vi "Test Overrides Has Case Structure Removed.vi"(8 "error in (no error)":errorcluster, 11 "Test Case In":refnum<class "Pure Mock Class Generator Test.lvclass">) -> (0 "error out":errorcluster, 3 "Test Case Out":refnum<class "Pure Mock Class Generator Test.lvclass">)   [LabVIEW 2020, in "Pure Mock Class Generator Test.lvclass"]
uses:
  Pure Mock Class Generator Test.lvclass
  C:/Program Files (x86)/National Instruments/LabVIEW 2020/vi.lib/Astemes/LUnit/Test Case.lvclass
  <vilib>/Utility/traverseref.llb/TRef TravTarget.ctl
  <vilib>/Astemes/LUnit/Test Case.lvclass/Test Case.ctl
  <vilib>/Astemes/LUnit/Append Fail Result.vi
  <vilib>/Astemes/LUnit/Append Pass Result.vi
  <vilib>/Utility/traverseref.llb/VI Scripting - Traverse.lvlib
  <vilib>/Astemes/LUnit/Test Case.lvclass
  source/Scripting/Pure Mock Class Generator/Pure Mock Class Generator.lvclass
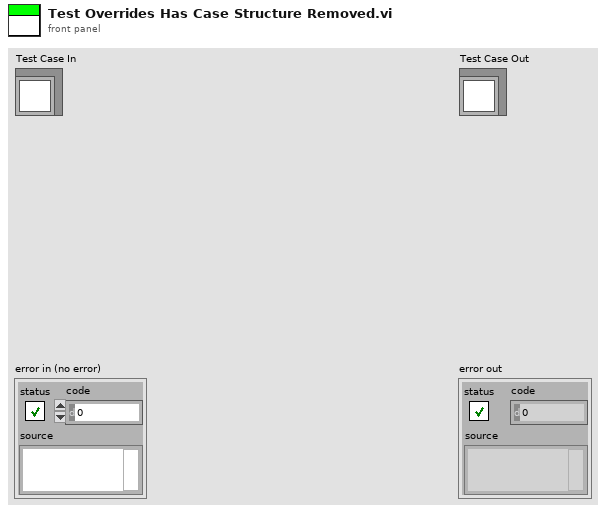
[diagram p1: front panel]
types:
  T1 = typedef "TRef TravTarget.ctl" = enum16{"FP", "BD", "Other"}
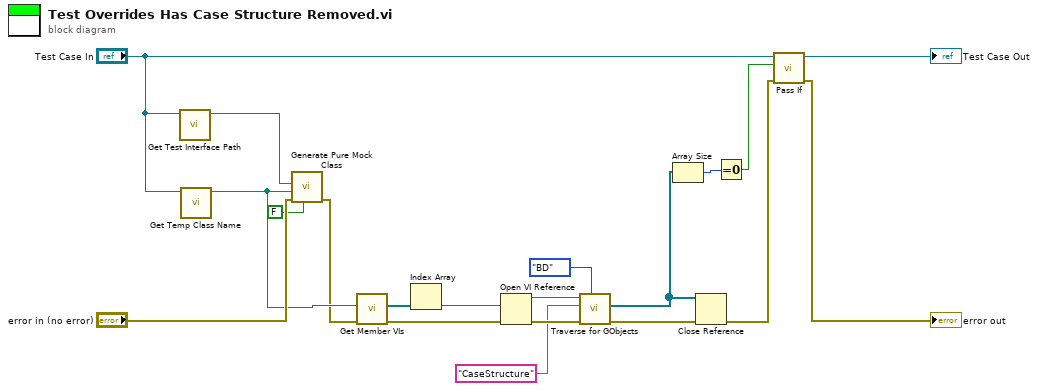
[diagram p0: block diagram]
diagram:
  n1 = call "Get Test Interface Path.vi"("Mock Class Generator Test in"="Test Case In") -> ("Test Class Path"=w16:path)  [unwired: 10 in]
  n2 = call "Get Temp Class Name.vi"("Mock Class Generator Test in"="Test Case In") -> ("Test Class Path"=w15:path)  [unwired: 10 in]
  n3 = call "Generate Pure Mock Class.vi"("Add to lvproj?"=FALSE, "error in (no error)"="error in (no error)", "Destination Class Path"=w15, "Source Class Path"=w16) -> ("error out"=w14:errorcluster)  [unwired: 7 in]
  n4 = call "Get Member VIs.vi"("error in (no error)"=w14, "Test Class Path"=w15) -> ("error out"=w13:errorcluster, "Array"=w12:path[])  [unwired: 8 in]
  n5 = Index Array(array=w12) -> (element=w10:path)  [unwired: 1 in]
  n6 = Open VI Reference(vi path=w10, error in (no error)=w13) -> (vi reference=w9:refnum<vi>, error out=w11:errorcluster)  [unwired: 4 in]
  n7 = call <vilib>:"Traverse for GObjects.vi"("Traverse Target"=TRef_TravTarget."BD", "error in (no error)"=w11, "Class Name"="CaseStructure", "VI Refnum"=w9) -> ("error out"=w6:errorcluster, "References"=w2:refnum<vi>[])  [unwired: 4 in, 2 out]
  n8 = Array Size(array=w2) -> (size(s)=w5:i32)
  n9 = Close Reference(reference=w2, error in (no error)=w6) -> (error out=w3:errorcluster)
  n10 = Equal To 0?(x=w5) -> (x = 0?=w4:bool)
  n11 = call <vilib>:"Pass If.vi"("error in (no error)"=w3, "Pass?"=w4, "LUnit Test Case In"="Test Case In") -> ("error out"=→"error out":errorcluster, "LUnit Test Case Out"=→"Test Case Out":refnum<class "Pure Mock Class Generator Test.lvclass">)  [unwired: 7 in]
